vi "Motic Get Exposure Range.vi"(8 "error in (no error)":errorcluster, 11 "camera":i32) -> (0 "error out":errorcluster, 1 "range max":sgl, 2 "range min":sgl, 3 "camera out":i32)   [LabVIEW 2012, in "MoticApi.lvlib"]
doc: "MOTICAPI bool Motic_GetExposureRange(MUCam_Handle camera, float *min, float *max);"
uses:
  MoticApi.lvlib
  MoticApi.dll
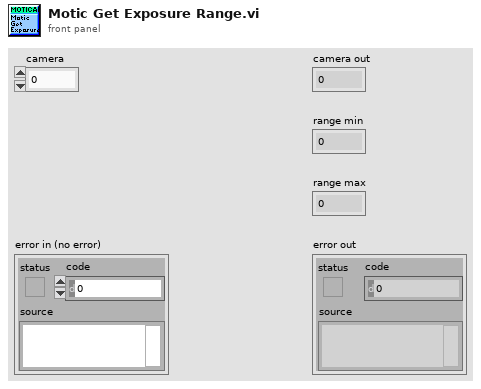
[diagram p1: front panel]
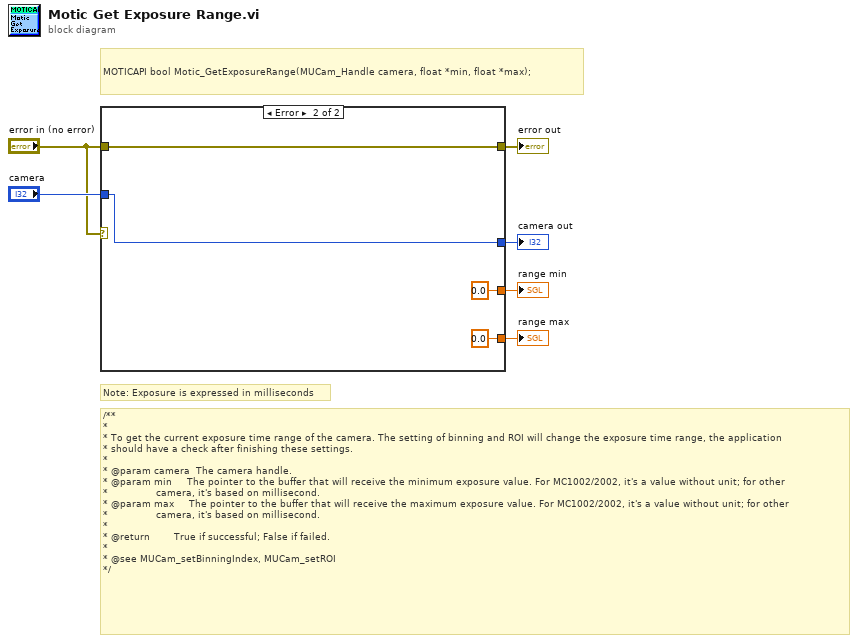
[diagram p0: block diagram]
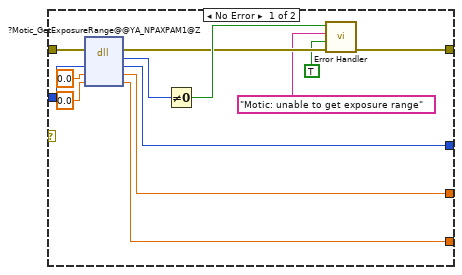
[diagram p2: hidden frame]
diagram:
  # "/**\n*\n* To get the current exposure time range of the camera. The setting of binning and ROI will change the exposure time range, the application\n* should have a check after finishing these settings.\n*\n* @param camera  The camera handle.\n* @param min     The pointer to the buffer that will receive the minimum exposure value. For MC1002/2002, it's a value without unit; for other\n*                camera, it's based on millisecond.\n* @param max     The pointer to the buffer that will receive the maximum exposure value. For MC1002/2002, it's a value without unit; for other\n*                camera, it's based on millisecond.\n*\n* @return        True if successful; False if failed.\n*\n* @see MUCam_setBinningIndex, MUCam_setROI\n*/"
  # "Note: Exposure is expressed in milliseconds"
  # "MOTICAPI bool Motic_GetExposureRange(MUCam_Handle camera, float *min, float *max);"
  n1 = case shown="Error" "error in (no error)" {
    tunnel: "camera" -> [w19 w22]
    tunnel: [w18 w22] -> w5
    tunnel: [w16 sgl 0.0 ("range min")] -> w4
    tunnel: [w14 sgl 0.0 ("range max")] -> w3
    tunnel: "error in (no error)" -> [w13 w23]
    tunnel: [w12 w23] -> w2
    frame No Error {
      n2 = dll-call lib="C:/Users/TTS-Digital/Desktop/MoticApi/MoticApi_git/MoticApi/MoticApi.*" fn="?Motic_GetExposureRange@@YA_NPAXPAM1@Z"(error in=w13, "camera"=w19, "range min"=sgl 0.0, "range max"=sgl 0.0) -> (error out=w10:errorcluster, w9:u8, "camera"=w18:i32, "range min"=w16:sgl, "range max"=w14:sgl)  [unwired: 2 in, 1 out]
      n3 = Not Equal To 0?(x=w9) -> (x != 0?=w11:bool)
      n4 = call "Error Handler.vi"("error in (no error)"=w10, "Is warning?"=TRUE, "Error message"="Motic: unable to get exposure range", "Function return"=w11) -> ("error out"=w12:errorcluster)  [unwired: 7 in]
    }
    frame Error {
    }
  }
  "camera out" <- w5
  "range min" <- w4
  "range max" <- w3
  "error out" <- w2
